vi "ROS_Topic_Write_Primitive.vi"(2 "Msg in":string, 3 "ROS in":T1={"topic port"=0, "Node"="", "topic"="", "type"="", "node port"=0, "error "={"status"=FALSE, "code"=0, "source"=""}, "Direction"=enum."Node", "Update (ms)"=1, "FIFO size"=1}) -> (1 "ROS out":T1={"topic port"=0, "Node"="", "topic"="", "type"="", "node port"=0, "error "={"status"=FALSE, "code"=0, "source"=""}, "Direction"=enum."Node", "Update (ms)"=1, "FIFO size"=1})   [LabVIEW 2012]
doc: "Writes the data to background server when publishing data or sending service calls. Implemented in ROS_Topic_Write and ROS_Topic_Write_Continuous."
uses:
  <userlib>/ROS for LabVIEW Software/ROS/Code/SubVIs/_ROSControl.ctl
  <userlib>/ROS for LabVIEW Software/ROS/Code/SubVIs/_ROSDirection.ctl
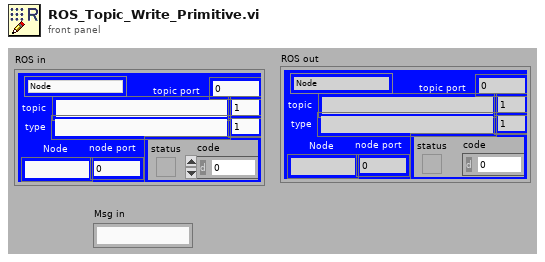
[diagram p1: front panel]
types:
  T1 = typedef "_ROSControl.ctl" = cluster{"topic port":u16, "Node":string, "topic":string, "type":string, "node port":u16, "error ":errorcluster, "Direction":T2, "Update (ms)":u16, "FIFO size":u16}
  T2 = typedef "_ROSDirection.ctl" = enum16{"Node", "Publisher", "Subscriber", "ServiceClient", "ServiceProvider"}
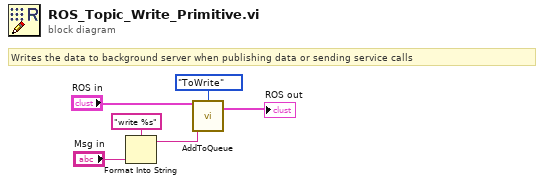
[diagram p0: block diagram]
diagram:
  # "Writes the data to background server when publishing data or sending service calls"
  n1 = Format Into String(format string="write %s" ("name (unnamed)"), "Msg in") -> (resulting string=w2:string)  [unwired: 2 in, 1 out]
  n2 = call <userlib>:"AddToQueue.vi"("Cmd"=w2, "ROS"="ROS in", "Type"=enum16{"topic", "node", "ToFIFO", "ToWrite"}."ToWrite") -> ("ROS out"=→"ROS out":T1)  [unwired: 2 in]
